vi "TRITON_SOLENOID_CONTROL_EXAMPLE.vi"() -> ()   [LabVIEW 2009]
panel:
  out "XY Graph":cluster{dbl[], dbl[]}(graph)
  out "Elapsed Time[s]":dbl
  out "Field [T]":dbl
  in  "STOP":bool
  out "Command String":string
  in  "Target Field":dbl
  in  "stop":bool
  in  "Time [min]":dbl
  in  "Rate [T / min]":dbl
  in  "Sweep Mode":enum16{"RATE", "TIME", "ASAP"}(ring)
  out "error out 2":errorcluster
  out "RI Response":string
  out "error out":errorcluster
  out "Connection Open":bool
  in  "error in (no error)":errorcluster
  in  "Open Connection":bool
  in  "Timeout":i32=10000
  in  "Remote Port":i32=33576
  in  "IP Address":string
  in  "Bytes to Read":i32=5000
  in  "Mode":T1(ring)=enum."Immediate"
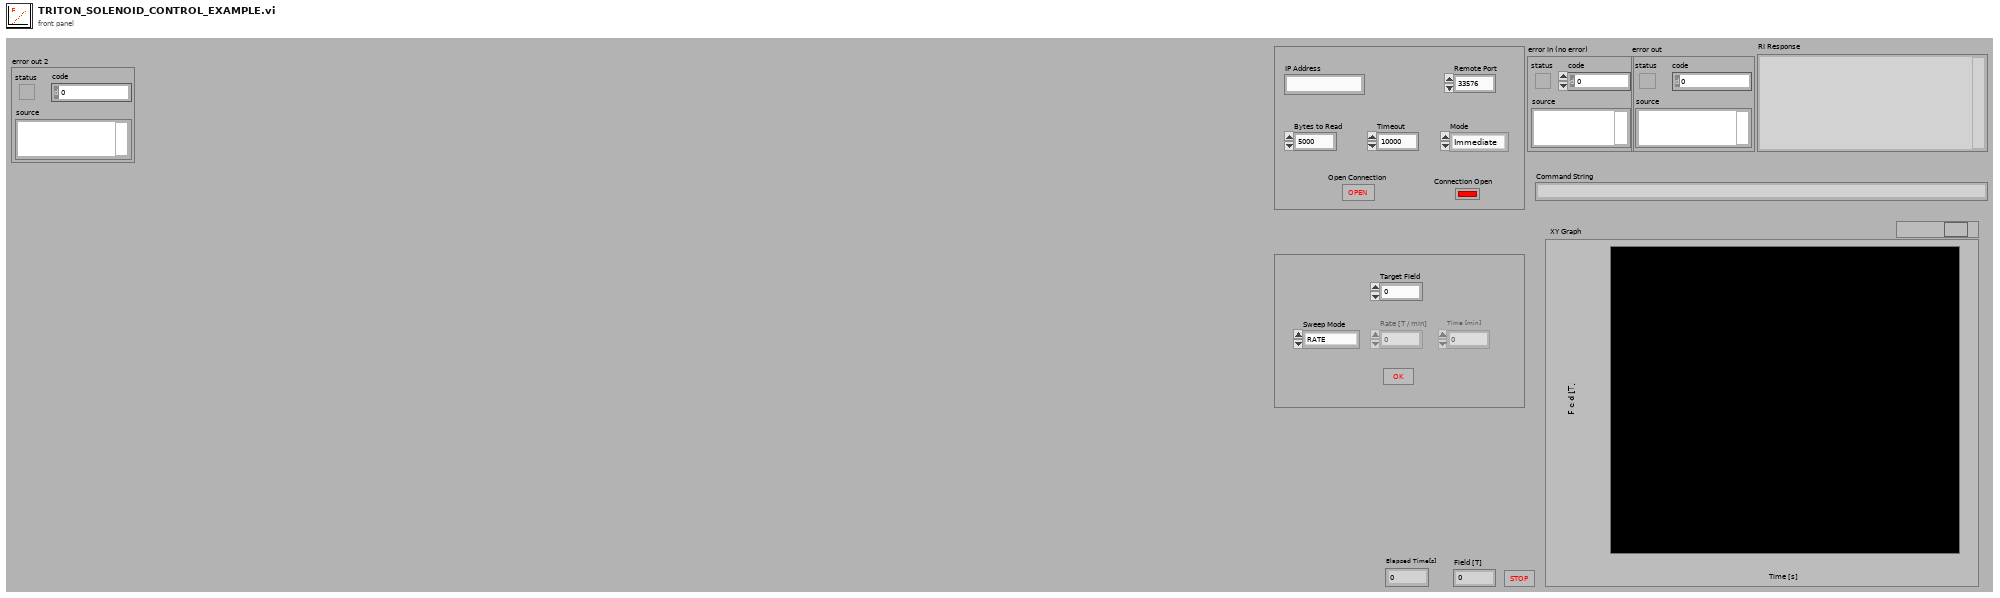
[diagram p1: front panel]
types:
  T1 = enum16{"Standard", "Buffered", "CRLF", "Immediate"}
  T2 = cluster{"Mode":enum16{"Standard", "Buffered", "CRLF", "Immediate"}, "Bytes to Read":i32, "IP Address":string, "Remote Port":i32, "Timeout":i32}
  T3 = cluster{"Mode":enum16{"Standard", "Buffered", "CRLF", "Immediate"}, "Bytes to Read":i32, "IP Address":string, "Remote Port":i32, "Timeout":i32, "connection ID":refnum<k5>}
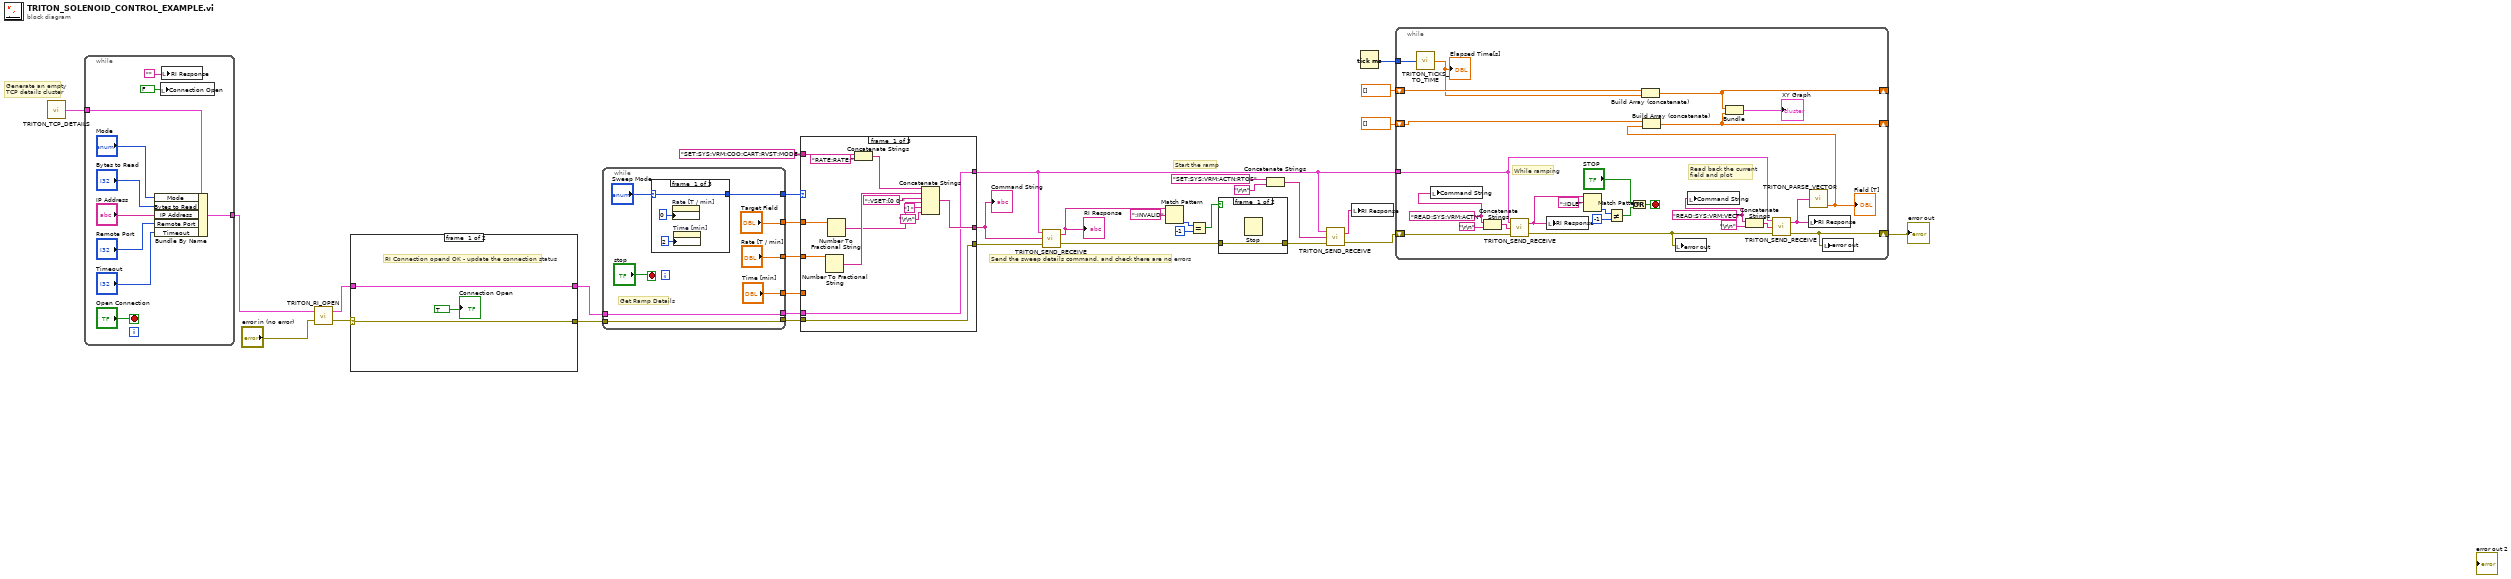
[diagram p0: block diagram]
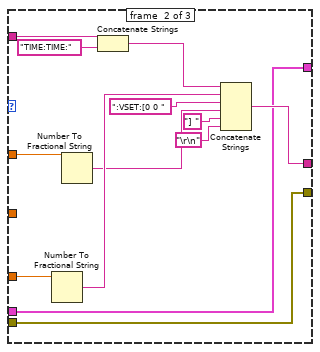
[diagram p3: hidden frame]
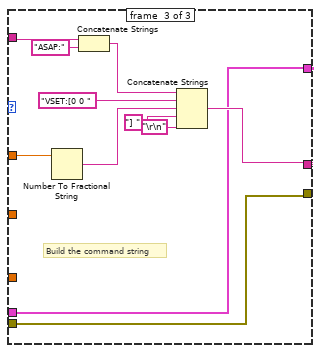
[diagram p4: hidden frame]
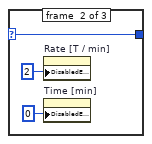
[diagram p5: hidden frame]
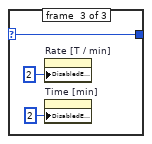
[diagram p6: hidden frame]
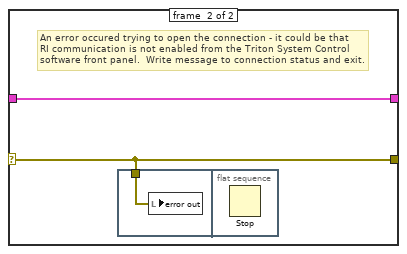
[diagram p7: hidden frame]
diagram:
  # "Start the ramp"
  # "Send the sweep details command, and check there are no errors"
  # "Generate an empty\nTCP details cluster"
  n1 = call "TRITON_TCP_DETAILS.vi"() -> ("Cluster"=w33:T2)
  n2 = while {
    tunnel: w33 -> [w42]
    tunnel: [w34] -> w32
    stop <- "Open Connection" stop-if-true
    n3 = Bundle By Name(cluster=w42, "Mode"="Mode", "Bytes to Read"="Bytes to Read", "IP Address"="IP Address", "Remote Port"="Remote Port", "Timeout"="Timeout") -> (w34:T2)
    n4 = local write "Connection Open"(FALSE ("Connection Open")) -> ()
    n5 = local write "RI Response"("") -> ()
  }
  n6 = call "TRITON_RI_OPEN.vi"("error in (no error)"="error in (no error)", "Cluster"=w32) -> ("error out"=w30:errorcluster, "output cluster"=w29:T3)
  n7 = case shown="Error" w30 {
    selector: w30 -> [w45 w47]
    tunnel: w29 -> [w46 w48]
    tunnel: [w46 w48] -> w27
    tunnel: [w45 w47] -> w28
    frame #0 {
      # "RI Connection opend OK - update the connection status"
      "Connection Open" <- TRUE ("Connection Open")
    }
    frame #1 {
      # "An error occured trying to open the connection - it could be that\nRI communication is not enabled from the Triton System Control\nsoftware front panel.  Write message to connection status and exit."
      n8 = flat-sequence {
        tunnel: w47 -> [w49]
        frame #0 {
          n9 = local write "error out"(w49) -> ()
        }
        frame #1 {
          n10 = Stop() -> ()  [unwired: 1 in]
        }
      }
    }
  }
  n11 = while {
    tunnel: [w55] -> w26
    tunnel: ["Target Field"] -> w25
    tunnel: ["Rate [T / min]"] -> w24
    tunnel: ["Time [min]"] -> w23
    tunnel: w28 -> [w51]
    tunnel: w27 -> [w50]
    tunnel: [w51] -> w21
    tunnel: [w50] -> w22
    stop <- "stop" stop-if-true
    # "Get Ramp Details"
    n12 = case shown="\"ASAP\"" "Sweep Mode" {
      selector: "Sweep Mode" -> [w58 w61 w64]
      tunnel: [w58 w61 w64] -> w55
      frame #0 {
        n13 = property on="Rate [T / min]" class="DigNum (strict)"("DisabledEnum"=0) -> ()  [unwired: 2 in, 2 out]
        n14 = property on="Time [min]" class="DigNum (strict)"("DisabledEnum"=2) -> ()  [unwired: 2 in, 2 out]
      }
      frame #1 {
        n15 = property on="Rate [T / min]" class="DigNum (strict)"("DisabledEnum"=2) -> ()  [unwired: 2 in, 2 out]
        n16 = property on="Time [min]" class="DigNum (strict)"("DisabledEnum"=0) -> ()  [unwired: 2 in, 2 out]
      }
      frame #2 {
        n17 = property on="Rate [T / min]" class="DigNum (strict)"("DisabledEnum"=2) -> ()  [unwired: 2 in, 2 out]
        n18 = property on="Time [min]" class="DigNum (strict)"("DisabledEnum"=2) -> ()  [unwired: 2 in, 2 out]
      }
    }
  }
  n19 = case shown="\"ASAP\"" w26 {
    tunnel: w25 -> [w76 w89 w101]
    tunnel: w24 -> [w77 _ _]
    tunnel: w23 -> [_ w90 _]
    tunnel: w22 -> [w69 w82 w95]
    tunnel: w21 -> [w68 w81 w94]
    tunnel: "SET:SYS:VRM:COO:CART:RVST:MODE:" -> [w79 w92 w103]
    tunnel: [w70 w83 w96] -> w18
    tunnel: [w69 w82 w95] -> w4
    tunnel: [w68 w81 w94] -> w19
    frame #0 {
      n20 = Number To Fractional String(number=w77) -> (F-format string=w72:string)  [unwired: 3 in]
      n21 = Number To Fractional String(number=w76) -> (F-format string=w71:string)  [unwired: 3 in]
      n22 = Concatenate Strings(w79, "RATE:RATE:") -> (w73:string)
      n23 = Concatenate Strings(w73, w72, ":VSET:[0 0 ", w71, "] ", "\r\n") -> (w70:string)
    }
    frame #1 {
      n24 = Number To Fractional String(number=w90) -> (F-format string=w87:string)  [unwired: 3 in]
      n25 = Number To Fractional String(number=w89) -> (F-format string=w85:string)  [unwired: 3 in]
      n26 = Concatenate Strings(w92, "TIME:TIME:") -> (w88:string)
      n27 = Concatenate Strings(w88, w87, ":VSET:[0 0 ", w85, "] ", "\r\n") -> (w83:string)
    }
    frame #2 {
      # "Build the command string"
      n28 = Number To Fractional String(number=w101) -> (F-format string=w97:string)  [unwired: 3 in]
      n29 = Concatenate Strings(w103, "ASAP:") -> (w98:string)
      n30 = Concatenate Strings(w98, "VSET:[0 0 ", w97, "] ", "\r\n") -> (w96:string)
    }
  }
  "Command String" <- w18
  n31 = call "TRITON_SEND_RECEIVE.vi"("error in (no error)"=w19, "Command String"=w18, "Communication Cluster"=w4) -> ("error out"=w12:errorcluster, "Response String"=w17:string)
  "RI Response" <- w17
  n32 = Match Pattern(string=w17, regular expression=":INVALID") -> (offset past match=w15:i32)  [unwired: 1 in, 3 out]
  n33 = Equal?(x=w15, y=-1) -> (x = y?=w13:bool)
  n34 = case shown="False" w13 {
    tunnel: w12 -> [w104 w105]
    tunnel: [w104 w105] -> w11
    frame #0 {
      n35 = Stop() -> ()  [unwired: 1 in]
    }
    frame #1 {
    }
  }
  n36 = Concatenate Strings("SET:SYS:VRM:ACTN:RTOS" ("Command String"), "\r\n") -> (w8:string)
  n37 = call "TRITON_SEND_RECEIVE.vi"("error in (no error)"=w11, "Command String"=w8, "Communication Cluster"=w4) -> ("error out"=w6:errorcluster, "Response String"=w7:string)
  n38 = local write "RI Response"(w7) -> ()
  n39 = Tick Count (ms)() -> (millisecond timer value=w3:u32)
  n40 = while {
    shift-right: [w107] -> w5
    shift-left: w6 -> [w127]
    tunnel: w4 -> [w118]
    tunnel: w3 -> [w121]
    shift-right: [w112] -> _
    shift-left: dbl[] [] -> [w116]
    shift-right: [w111] -> _
    shift-left: dbl[] [] -> [w113]
    stop <- w126 stop-if-true
    w109 = "READ:SYS:VRM:VECT" ("regular expression")
    w110 = "READ:SYS:VRM:ACTN" ("regular expression")
    # "Read back the current\nfield and plot"
    # "While ramping"
    n41 = call "TRITON_TICKS_TO_TIME.vi"("Initial millisecond timer value"=w121) -> ("Elapsed Time in Seconds"=w115:dbl)
    "Elapsed Time[s]" <- w115
    n42 = local write "Command String"(w110) -> ()
    n43 = Concatenate Strings(w110, "\r\n") -> (w122:string)
    n44 = call "TRITON_SEND_RECEIVE.vi"("error in (no error)"=w127, "Command String"=w122, "Communication Cluster"=w118) -> ("error out"=w106:errorcluster, "Response String"=w128:string)
    n45 = local write "RI Response"(w128) -> ()
    n46 = Match Pattern(string=w128, regular expression=":IDLE") -> (offset past match=w130:i32)  [unwired: 1 in, 3 out]
    n47 = Not Equal?(x=w130, y=-1) -> (x != y?=w125:bool)
    n48 = Or(x="STOP", y=w125) -> (x .or. y?=w126:bool)
    n49 = Build Array (concatenate)(w116, w115) -> (w112:dbl[])
    n50 = local write "error out"(w106) -> ()
    n51 = local write "Command String"(w109) -> ()
    n52 = Concatenate Strings(w109, "\r\n") -> (w120:string)
    n53 = call "TRITON_SEND_RECEIVE.vi"("error in (no error)"=w106, "Command String"=w120, "Communication Cluster"=w118) -> ("error out"=w107:errorcluster, "Response String"=w117:string)
    n54 = local write "RI Response"(w117) -> ()
    n55 = call "TRITON_PARSE_VECTOR.vi"("String"=w117) -> ("Z"=w114:dbl)  [unwired: 2 out]
    "Field [T]" <- w114
    n56 = Build Array (concatenate)(w113, w114) -> (w111:dbl[])
    n57 = Bundle(w112, w111) -> (→"XY Graph":cluster{dbl[], dbl[]})  [unwired: 1 in]
    n58 = local write "error out"(w107) -> ()
  }
  "error out" <- w5
